vi "CamGetExpo.vi"(8 "error in (no error)":errorcluster, 11 "hCam":i16) -> (0 "error in (no error) 2":errorcluster, 2 "exposure":u32, 3 "hCam out":i16)   [LabVIEW 2021]
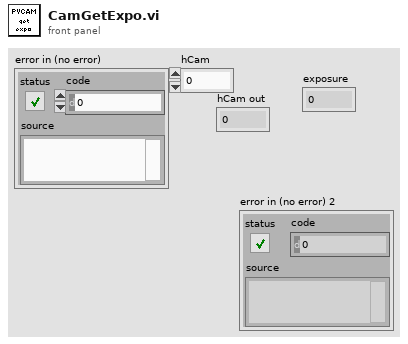
[diagram p1: front panel]
types:
  T1 = enum16{"ATTR_CURRENT", "ATTR_COUNT", "ATTR_TYPE", "ATTR_MIN", "ATTR_MAX", "ATTR_DEFAULT", "ATTR_INCREMENT", "ATTR_ACCESS", "ATTR_AVAIL"}
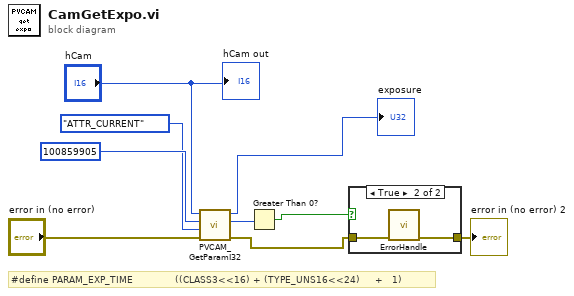
[diagram p0: block diagram]
diagram:
  # "#define PARAM_EXP_TIME              ((CLASS3<<16) + (TYPE_UNS16<<24)     +   1)"
  n1 = call "PVCAM_GetParamI32.vi"("error in (no error)"="error in (no error)", "param_attrib"=T1."ATTR_CURRENT", "param_id"=u32 100859905, "hCam"="hCam") -> ("error out"=w4:errorcluster, "return type"=w5:i16, "param_value"=→"exposure":u32)  [unwired: 5 in]
  n2 = Greater Than 0?(x=w5) -> (x > 0?=w2:bool)
  n3 = case shown="True" w2 {
    tunnel: w4 -> [w10 w12]
    tunnel: [w10 w11] -> w3
    frame False {
    }
    frame True {
      n4 = call "ErrorHandle.vi"("error in (no error)"=w12) -> ("error in (no error) 2"=w11:errorcluster)  [unwired: 10 in]
    }
  }
  "error in (no error) 2" <- w3
  "hCam out" <- "hCam"
